vi "Get Macro String.vi"(8 "error in (no error)":errorcluster) -> (0 "error out":errorcluster)   [LabVIEW 2013, in "JKI State Machine API - Tests.lvlib"]
uses:
  JKI State Machine API - Tests.lvlib
  <vilib>/addons/_JKI Toolkits/Caraya/classes/Assert/Assert.lvclass
  <vilib>/addons/_JKI Toolkits/Caraya/classes/Test/Test.lvclass
  source/JKI SM/JKI SM.lvclass
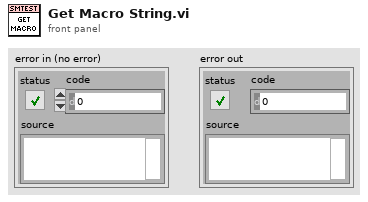
[diagram p1: front panel]
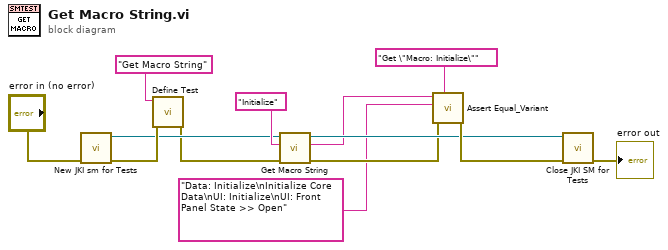
[diagram p0: block diagram]
diagram:
  n1 = call "New JKI sm for Tests.vi"("error in (no error)"="error in (no error)") -> ("error out"=w13:errorcluster, "JKI SM out"=w6:refnum<class "JKI SM.lvclass">)  [unwired: 9 in]
  n2 = call <vilib>:"Define Test.vi"("error in (no error)"=w13, "Label (VI Title)"="Get Macro String") -> ("error out"=w4:errorcluster)  [unwired: 9 in]
  n3 = call "Get Macro String.vi"("error in (no error)"=w4, "Macro Name"="Initialize", "JKI SM in"=w6) -> ("error out"=w3:errorcluster, "Macro String"=w1:string, "JKI SM out"=w5:refnum<class "JKI SM.lvclass">)  [unwired: 6 in]
  n4 = call <vilib>:"Assert Equal_Variant.vi"("Label"="Get \"Macro: Initialize\"", "error in (no error)"=w3, "Y"="Data: Initialize\nInitialize Core Data\nUI: Initialize\nUI: Front Panel State >> Open" ("Macro String"), "X"=w1) -> ("error out"=w10:errorcluster)  [unwired: 7 in]
  n5 = call "Close JKI SM for Tests.vi"("error in (no error)"=w10, "JKI SM in"=w5) -> ("error out"=→"error out":errorcluster)  [unwired: 9 in]
